vi "arrange VI.vi"(6 "Show FP (F)":bool, 7 "FP (T)":bool=TRUE, 8 "error in":errorcluster, 11 "VI in":refnum<vi>) -> (0 "error out":errorcluster, 3 "VI out":refnum<vi>)   [LabVIEW 2020]
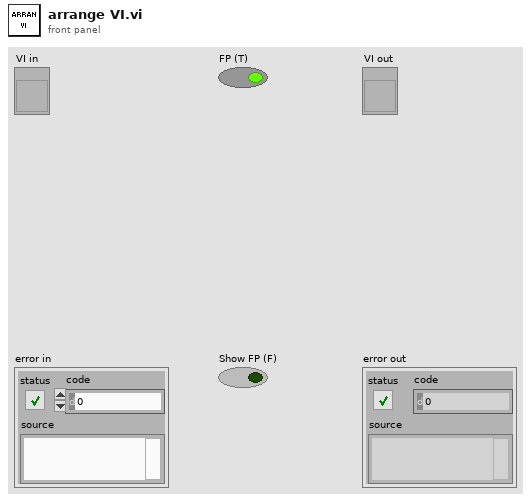
[diagram p1: front panel]
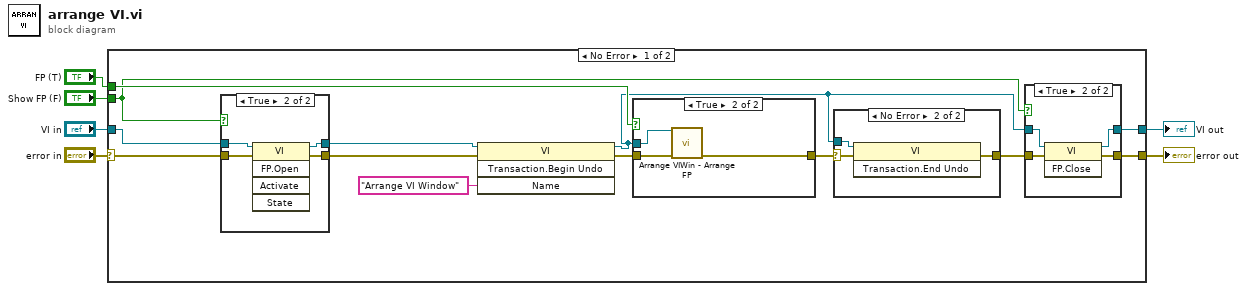
[diagram p0: block diagram]
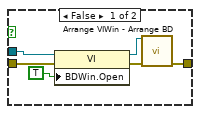
[diagram p4: hidden frame]
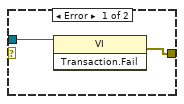
[diagram p5: hidden frame]
diagram:
  n1 = case shown="No Error" "error in" {
    selector: "error in" -> [w11 w46]
    tunnel: [w19 w46] -> w6
    tunnel: [w17 w47] -> w5
    tunnel: "Show FP (F)" -> [w10 _]
    tunnel: "FP (T)" -> [w15 _]
    tunnel: "VI in" -> [w14 w47]
    frame No Error {
      n2 = case shown="True" w10 {
        tunnel: [w21 w25] -> w16
        tunnel: [w20 w24] -> w7
        tunnel: w14 -> [w21 w23]
        tunnel: w11 -> [w20 w22]
        frame False {
        }
        frame True {
          n3 = invoke class="VI" method="FP.Open"(reference=w23, error in=w22) -> (reference out=w25:refnum<vi>, error out=w24:errorcluster)  [unwired: 3 in, 3 out]
        }
      }
      n4 = invoke class="VI" method="Transaction.Begin Undo"(reference=w16, error in=w7, "Name"="Arrange VI Window") -> (reference out=w9:refnum<vi>, error out=w12:errorcluster)  [unwired: 1 in, 2 out]
      n5 = case shown="True" w15 {
        tunnel: w12 -> [w35 w39]
        tunnel: [w37 w40] -> w13
        tunnel: w9 -> [w36 w38]
        frame False {
          n6 = property class="VI"(reference=w36, error in=w35, "BDWin.Open"=TRUE ("Block Diagram Window:Open")) -> (reference out=w32:refnum<vi>, error out=w33:errorcluster)
          n7 = call <resource>:"Arrange VIWin - Arrange BD.vi"("VI in"=w32, "error in"=w33) -> ("error out"=w37:errorcluster)  [unwired: 13 in]
        }
        frame True {
          n8 = call <resource>:"Arrange VIWin - Arrange FP.vi"("VI"=w38, "error in"=w39) -> ("error out"=w40:errorcluster)  [unwired: 13 in]
        }
      }
      n9 = case shown="No Error" w13 {
        selector: w13 -> [_ w43]
        tunnel: w9 -> [w41 w44]
        tunnel: [w42 w45] -> w18
        frame Error {
          n10 = invoke class="VI" method="Transaction.Fail"(reference=w41) -> (error out=w42:errorcluster)  [unwired: 2 in, 2 out]
        }
        frame No Error {
          n11 = invoke class="VI" method="Transaction.End Undo"(reference=w44, error in=w43) -> (error out=w45:errorcluster)  [unwired: 1 in, 2 out]
        }
      }
      n12 = case shown="True" w10 {
        tunnel: w9 -> [w27 w28]
        tunnel: [w27 w29] -> w17
        tunnel: w18 -> [w26 w31]
        tunnel: [w26 w30] -> w19
        frame False {
        }
        frame True {
          n13 = invoke class="VI" method="FP.Close"(reference=w28, error in=w31) -> (reference out=w29:refnum<vi>, error out=w30:errorcluster)  [unwired: 1 in, 1 out]
        }
      }
    }
    frame Error {
    }
  }
  "error out" <- w6
  "VI out" <- w5
